vi "Poll PSA Freq Lock.vi"(8 "error in (no error)":errorcluster, 10 "Time Target (s)":dbl=15.0 format="%#_13g", 11 "VISA resource":refnum<visa-resource-name>="PSA1") -> (0 "error out":errorcluster, 3 "Locked":bool)   [LabVIEW 2015]
panel:
  out "Elapsed Time to Reference Lock":u32(slide) scale=0.0..15.0
  out "Elapsed Time (s)":u32 format="%<%H:%M:%S>t"
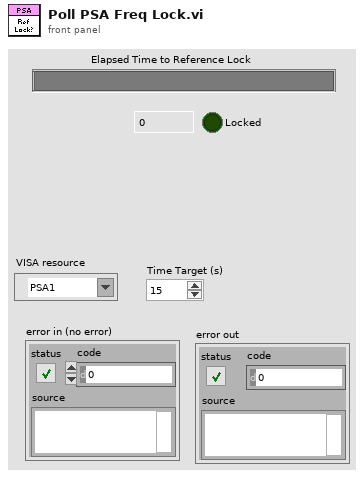
[diagram p1: front panel]
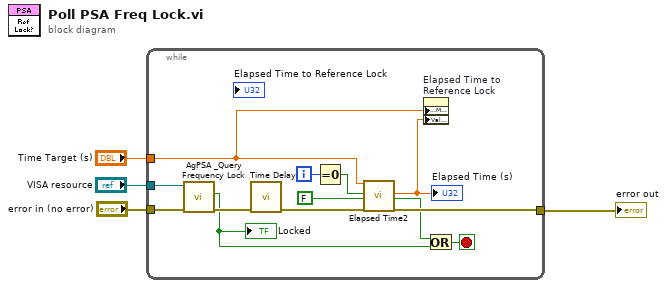
[diagram p0: block diagram]
diagram:
  n1 = while {
    tunnel: [w16] -> w1
    tunnel: "error in (no error)" -> [w9]
    tunnel: "VISA resource" -> [w8]
    tunnel: "Time Target (s)" -> [w6]
    i -> [w12]
    stop <- w13 stop-if-true
    n2 = call "AgPSA _Query Frequency Lock.vi"("error in (no error)"=w9, "VISA resource"=w8) -> ("error out"=w15:errorcluster, "Locked"=w7:bool)  [unwired: 7 in, 1 out]
    "Locked" <- w7
    n3 = call "Time Delay"("error in (no error)"=w15) -> ("error out"=w17:errorcluster)  [unwired: 10 in]
    n4 = Equal To 0?(x=w12) -> (x = 0?=w11:bool)
    n5 = call "Elapsed Time2"("Time Target (s)"=w6, "Reset"=w11, "Auto Reset"=FALSE, "error in (no error)"=w17) -> ("Elapsed Time (s)"=w5:dbl, "Time has Elapsed"=w14:bool, "error out"=w16:errorcluster)  [unwired: 8 in, 5 out]
    "Elapsed Time (s)" <- w5
    n6 = property on="Elapsed Time to Reference Lock" class="Slide (strict)"("Scale.Maximum"=w6, "Value"=w5) -> ()  [unwired: 2 in, 2 out]
    n7 = Or(x=w14, y=w7) -> (x .or. y?=w13:bool)
  }
  "error out" <- w1
